vi "Ball Fight.vi"() -> ()   [LabVIEW 2014]
panel:
  in  "?":bool
  in  "Computer?":bool=TRUE
  out "BOT":u8(slide)
  out "Player":u8(slide) scale=0.0..5.0
  out "力道":dbl(slide)
  in  "pok2":bool
  out "角度":dbl(knob)
  in  "aok2":bool
  out "cannonball 2":bool
  out "角度":dbl(knob) scale=0.0..1.5
  in  "aok1":bool
  out "Wind":dbl(slide) scale=-50.0..50.0
  out "力道":dbl(slide) scale=0.0..150.0
  in  "pok1":bool
  out "cannonball":bool
  # "Angle off?"
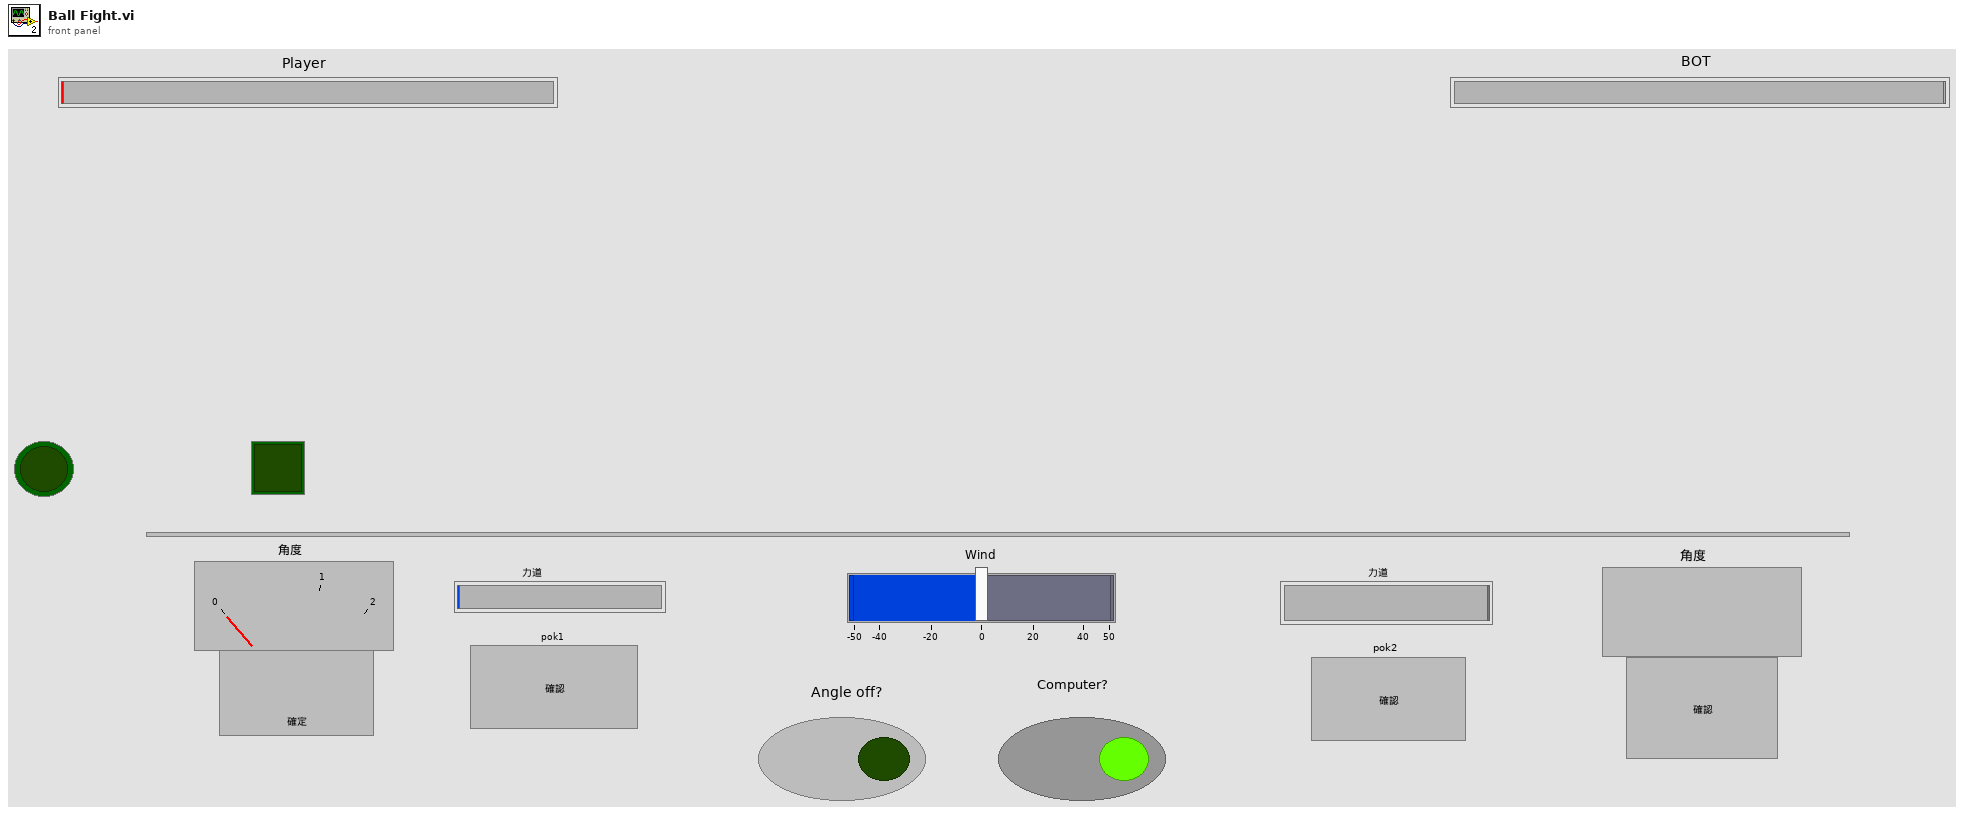
[diagram p1: front panel]
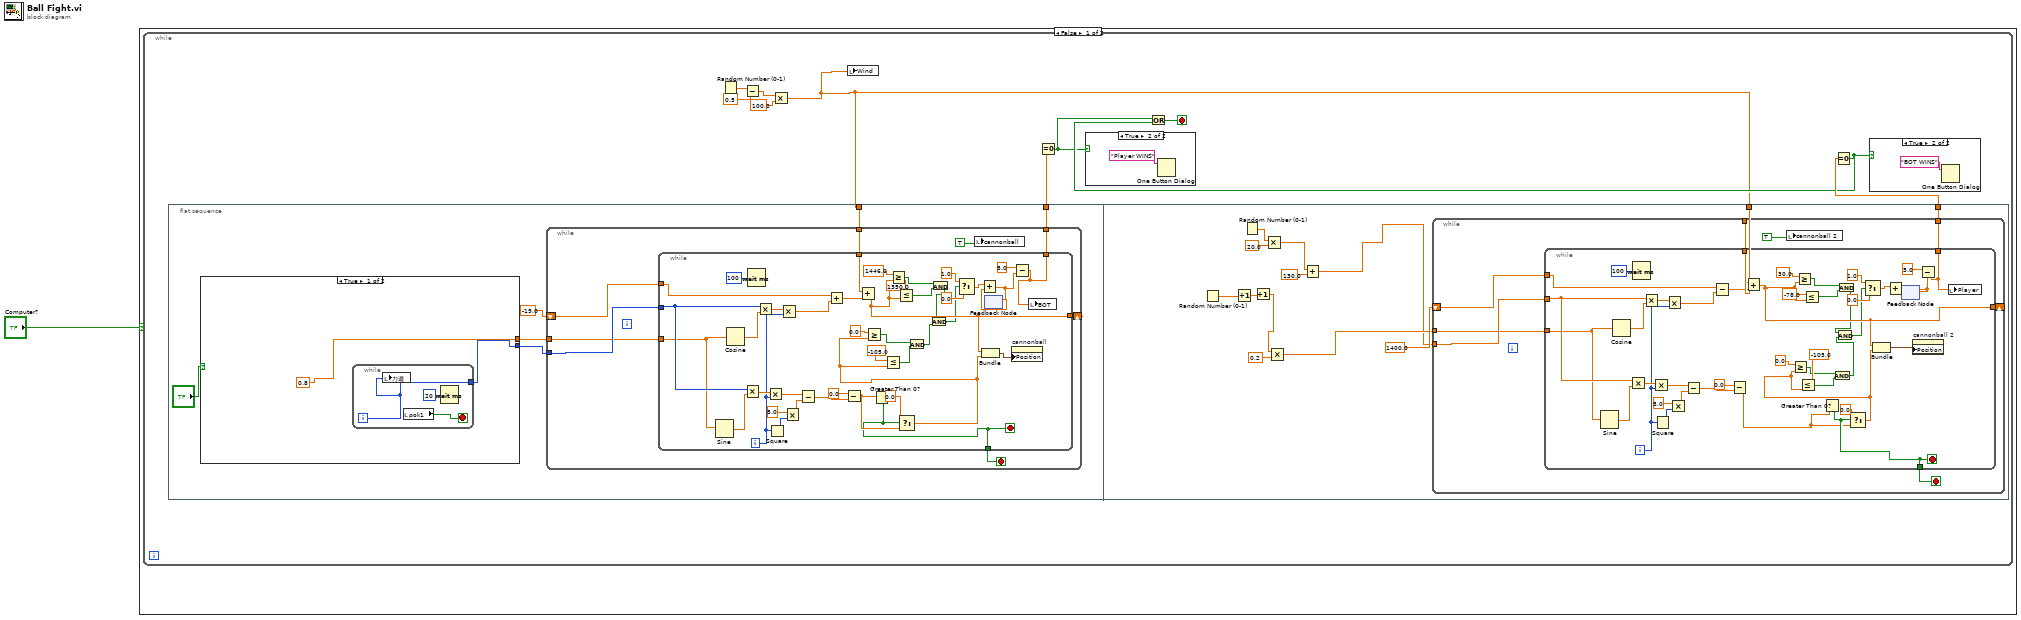
[diagram p0: block diagram]
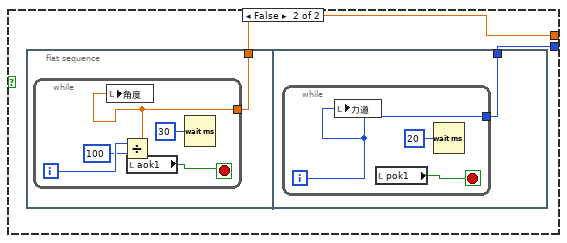
[diagram p4: hidden frame]
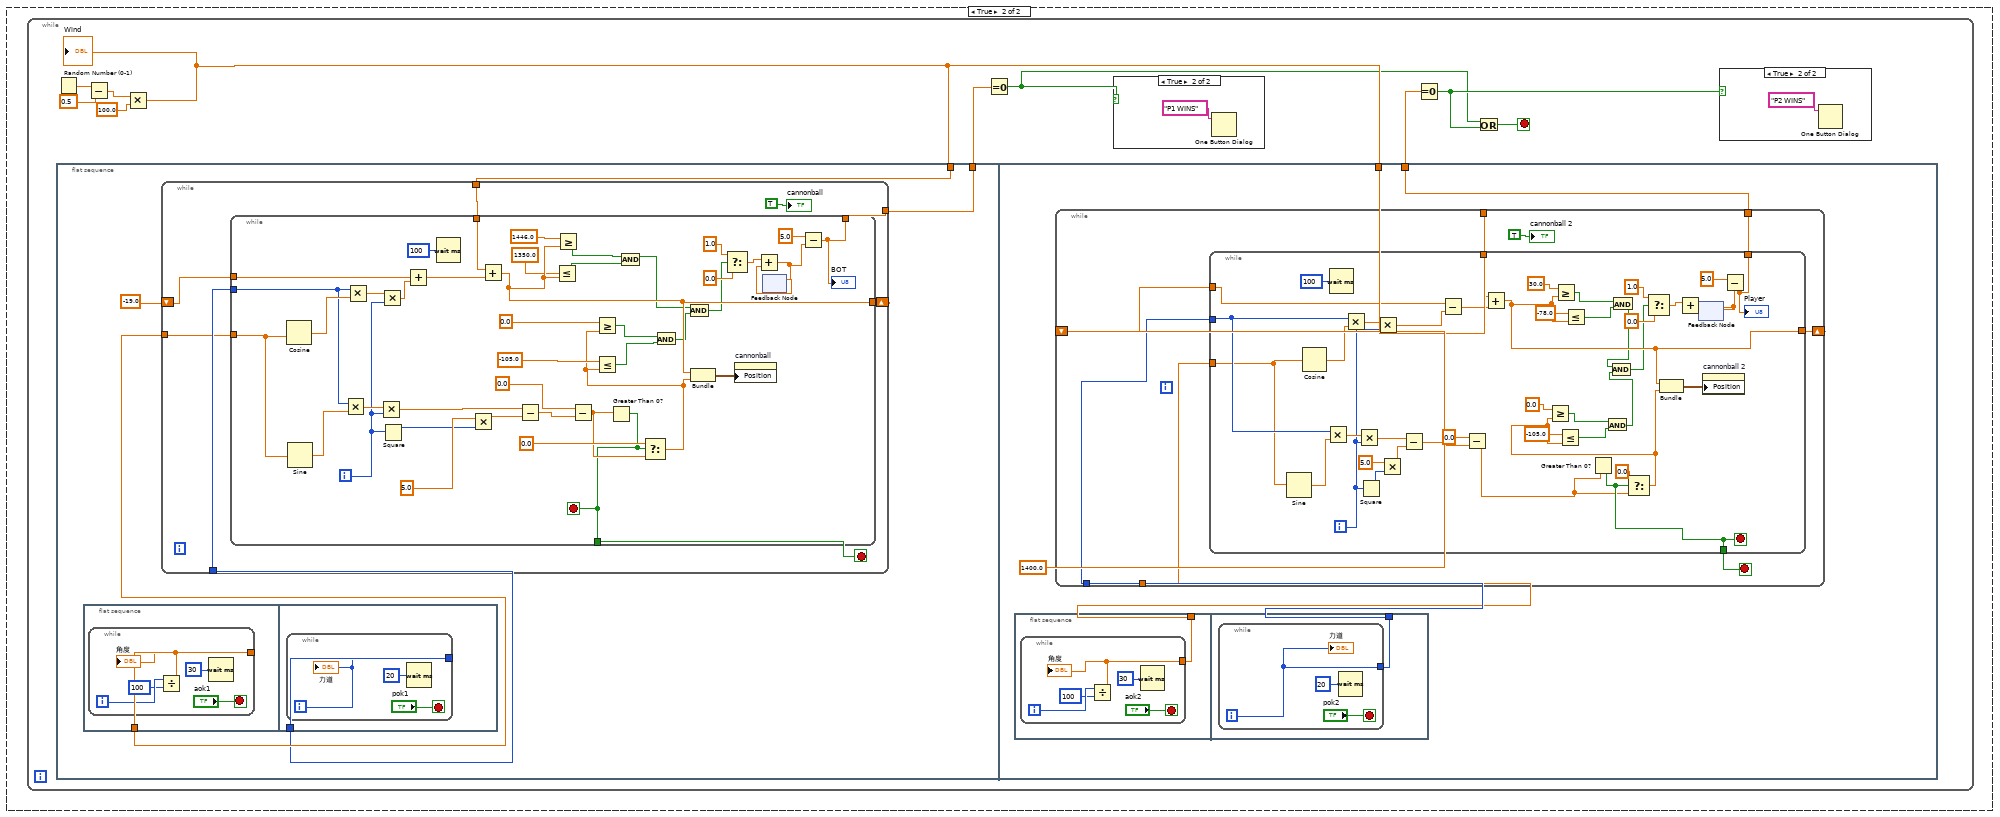
[diagram p5: hidden frame]
diagram:
  n1 = case shown="False" "Computer?" {
    frame False {
      n2 = while {
        stop <- w5 stop-if-true
        n3 = flat-sequence {
          tunnel: w2 -> [w18]
          tunnel: [w15] -> w7
          tunnel: w2 -> [w98]
          tunnel: [w97] -> w6
          frame #0 {
            n4 = case shown="True" "?" {
              tunnel: [0.8 w26] -> w17
              tunnel: [w21 w25] -> w16
              frame True {
                n5 = while {
                  tunnel: [w23] -> w21
                  i -> [w23]
                  stop <- w22 stop-if-true
                  n6 = local write "力道"(w23) -> ()
                  n7 = local read "pok1"() -> (w22:bool)
                  n8 = Wait (ms)(milliseconds to wait=u32 20) -> ()  [unwired: 1 out]
                }
              }
              frame False {
                n9 = flat-sequence {
                  tunnel: [w27] -> w26
                  tunnel: [w33] -> w25
                  frame #0 {
                    n10 = while {
                      tunnel: [w29] -> w27
                      i -> [w31]
                      stop <- w28 stop-if-true
                      n11 = Divide(x=w31, y=100) -> (x/y=w29:dbl)
                      n12 = local write "角度"(w29) -> ()
                      n13 = local read "aok1"() -> (w28:bool)
                      n14 = Wait (ms)(milliseconds to wait=u32 30) -> ()  [unwired: 1 out]
                    }
                  }
                  frame #1 {
                    n15 = while {
                      tunnel: [w35] -> w33
                      i -> [w35]
                      stop <- w34 stop-if-true
                      n16 = local write "力道"(w35) -> ()
                      n17 = local read "pok1"() -> (w34:bool)
                      n18 = Wait (ms)(milliseconds to wait=u32 20) -> ()  [unwired: 1 out]
                    }
                  }
                }
              }
            }
            n19 = while {
              shift-right: [w44] -> _
              shift-left: -19.0 -> [w43]
              tunnel: w16 -> [w42]
              tunnel: w18 -> [w40]
              tunnel: w17 -> [w39]
              tunnel: [w38] -> w15
              stop <- w41 stop-if-true
              n20 = while {
                tunnel: w42 -> [w72]
                tunnel: [w64] -> w44
                tunnel: w43 -> [w70]
                tunnel: [w69] -> w41
                tunnel: w40 -> [w67]
                tunnel: w39 -> [w66]
                tunnel: [w51] -> w38
                i -> [w79]
                stop <- w69 stop-if-true
                n21 = Sine(x=w66) -> (sin(x)=w83:dbl)
                n22 = Cosine(x=w66) -> (cos(x)=w86:dbl)
                n23 = Multiply(x=w72, y=w83) -> (x*y=w84:dbl)
                n24 = Wait (ms)(milliseconds to wait=u32 100) -> ()  [unwired: 1 out]
                n25 = Multiply(x=w72, y=w86) -> (x*y=w85:dbl)
                n26 = Multiply(x=w84, y=w79) -> (x*y=w82:dbl)
                n27 = Square(x=w79) -> (x^2=w80:i32)
                n28 = Multiply(x=w85, y=w79) -> (x*y=w71:dbl)
                n29 = Multiply(x=5.0, y=w80) -> (x*y=w78:dbl)
                n30 = Subtract(x=w82, y=w78) -> (x-y=w76:dbl)
                n31 = Add(x=w70, y=w71) -> (x+y=w68:dbl)
                n32 = Subtract(x=0.0, y=w76) -> (x-y=w73:dbl)
                n33 = Add(x=w67, y=w68) -> (x+y=w64:dbl)
                n34 = Greater Than 0?(x=w73) -> (x > 0?=w69:bool)
                n35 = Greater Or Equal?(x=1446.0, y=w64) -> (x >= y?=w62:bool)
                n36 = Less Or Equal?(x=1350.0, y=w64) -> (x <= y?=w61:bool)
                n37 = Select(t=0.0, s=w69, f=w73) -> (s? t:f=w45:dbl)
                n38 = Greater Or Equal?(x=0.0, y=w45) -> (x >= y?=w48:bool)
                n39 = Less Or Equal?(x=-105.0, y=w45) -> (x <= y?=w47:bool)
                n40 = And(x=w48, y=w47) -> (x .and. y?=w46:bool)
                n41 = And(x=w62, y=w61) -> (x .and. y?=w54:bool)
                n42 = And(x=w54, y=w46) -> (x .and. y?=w53:bool)
                n43 = Select(t=1.0, s=w53, f=0.0) -> (s? t:f=w58:dbl)
                n44 = Bundle(w64, "t"=w45) -> (w52:cluster{dbl, "t":dbl})  [unwired: 1 in]
                n45 = feedback #1() -> (w57:dbl)  [unwired: 1 in]
                n46 = Add(x=w58, y=w57) -> (x+y=w55:dbl)
                n47 = feedback-in #1(w55) -> ()
                n48 = property on="cannonball" class="Bool (strict)"("Position"=w52) -> ()  [unwired: 2 in, 2 out]
                n49 = Subtract(x=5.0, y=w55) -> (x-y=w51:dbl)
                n50 = local write "BOT"(w51) -> ()
              }
              n51 = local write "cannonball"(TRUE) -> ()
            }
          }
          frame #1 {
            n52 = Random Number (0-1)() -> (number: 0 to 1=w94:dbl)
            n53 = Increment(x=w94) -> (x+1=w93:dbl)
            n54 = Random Number (0-1)() -> (number: 0 to 1=w95:dbl)
            n55 = Increment(x=w93) -> (x+1=w91:dbl)
            n56 = Multiply(x=w95, y=20.0) -> (x*y=w87:dbl)
            n57 = Multiply(x=w91, y=0.2) -> (x*y=w90:dbl)
            n58 = Add(x=w87, y=130.0) -> (x+y=w88:dbl)
            n59 = while {
              shift-right: [w107] -> _
              shift-left: 1400.0 -> [w106]
              tunnel: w88 -> [w105]
              tunnel: w98 -> [w103]
              tunnel: w90 -> [w102]
              tunnel: [w101] -> w97
              stop <- w104 stop-if-true
              n60 = while {
                tunnel: w105 -> [w136]
                tunnel: [w121] -> w107
                tunnel: w106 -> [w134]
                tunnel: [w133] -> w104
                tunnel: w103 -> [w131]
                tunnel: w102 -> [w130]
                tunnel: [w108] -> w101
                i -> [w142]
                stop <- w133 stop-if-true
                n61 = Sine(x=w130) -> (sin(x)=w146:dbl)
                n62 = Cosine(x=w130) -> (cos(x)=w149:dbl)
                n63 = Multiply(x=w136, y=w146) -> (x*y=w147:dbl)
                n64 = Wait (ms)(milliseconds to wait=u32 100) -> ()  [unwired: 1 out]
                n65 = Multiply(x=w136, y=w149) -> (x*y=w148:dbl)
                n66 = Multiply(x=w147, y=w142) -> (x*y=w145:dbl)
                n67 = Square(x=w142) -> (x^2=w143:i32)
                n68 = Multiply(x=w148, y=w142) -> (x*y=w135:dbl)
                n69 = Multiply(x=5.0, y=w143) -> (x*y=w141:dbl)
                n70 = Subtract(x=w145, y=w141) -> (x-y=w139:dbl)
                n71 = Subtract(x=w134, y=w135) -> (x-y=w132:dbl)
                n72 = Subtract(x=0.0, y=w139) -> (x-y=w114:dbl)
                n73 = Add(x=w131, y=w132) -> (x+y=w121:dbl)
                n74 = Greater Or Equal?(x=30.0, y=w121) -> (x >= y?=w127:bool)
                n75 = Less Or Equal?(x=-78.0, y=w121) -> (x <= y?=w126:bool)
                n76 = Greater Than 0?(x=w114) -> (x > 0?=w133:bool)
                n77 = And(x=w127, y=w126) -> (x .and. y?=w112:bool)
                n78 = Select(t=0.0, s=w133, f=w114) -> (s? t:f=w110:dbl)
                n79 = Greater Or Equal?(x=0.0, y=w110) -> (x >= y?=w116:bool)
                n80 = Less Or Equal?(x=-105.0, y=w110) -> (x <= y?=w115:bool)
                n81 = And(x=w116, y=w115) -> (x .and. y?=w111:bool)
                n82 = And(x=w112, y=w111) -> (x .and. y?=w113:bool)
                n83 = Select(t=1.0, s=w113, f=0.0) -> (s? t:f=w123:dbl)
                n84 = Bundle(w121, "t"=w110) -> (w109:cluster{dbl, "t":dbl})  [unwired: 1 in]
                n85 = feedback #2() -> (w119:dbl)  [unwired: 1 in]
                n86 = Add(x=w123, y=w119) -> (x+y=w120:dbl)
                n87 = feedback-in #2(w120) -> ()
                n88 = property on="cannonball 2" class="Bool (strict)"("Position"=w109) -> ()  [unwired: 2 in, 2 out]
                n89 = Subtract(x=5.0, y=w119) -> (x-y=w108:dbl)
                n90 = local write "Player"(w108) -> ()
              }
              n91 = local write "cannonball 2"(TRUE) -> ()
            }
          }
        }
        n92 = Random Number (0-1)() -> (number: 0 to 1=w11:dbl)
        n93 = Subtract(x=w11, y=0.5) -> (x-y=w10:dbl)
        n94 = Multiply(x=w10, y=100.0) -> (x*y=w2:dbl)
        n95 = local write "Wind"(w2) -> ()
        n96 = Equal To 0?(x=w7) -> (x = 0?=w3:bool)
        n97 = case shown="True" w3 {
          frame False {
          }
          frame True {
            n98 = One Button Dialog(message="Player WINS" ("String")) -> ()  [unwired: 1 in, 1 out]
          }
        }
        n99 = Equal To 0?(x=w6) -> (x = 0?=w4:bool)
        n100 = Or(x=w3, y=w4) -> (x .or. y?=w5:bool)
        n101 = case shown="True" w4 {
          frame False {
          }
          frame True {
            n102 = One Button Dialog(message="BOT WINS" ("String")) -> ()  [unwired: 1 in, 1 out]
          }
        }
      }
    }
    frame True {
      n103 = while {
        stop <- w152 stop-if-true
        n104 = Random Number (0-1)() -> (number: 0 to 1=w159:dbl)
        n105 = flat-sequence {
          tunnel: w155 -> [w165]
          tunnel: [w162] -> w154
          tunnel: w155 -> [w229]
          tunnel: [w227] -> w153
          frame #0 {
            n106 = flat-sequence {
              tunnel: [w167] -> w164
              tunnel: [w173] -> w163
              frame #0 {
                n107 = while {
                  tunnel: [w169] -> w167
                  i -> [w170]
                  stop <- "aok1" stop-if-true
                  n108 = Divide(x=w170, y=100) -> (x/y=w169:dbl)
                  "角度" <- w169
                  n109 = Wait (ms)(milliseconds to wait=u32 30) -> ()  [unwired: 1 out]
                }
              }
              frame #1 {
                n110 = while {
                  tunnel: [w175] -> w173
                  i -> [w175]
                  stop <- "pok1" stop-if-true
                  n111 = Wait (ms)(milliseconds to wait=u32 20) -> ()  [unwired: 1 out]
                  "力道" <- w175
                }
              }
            }
            n112 = while {
              shift-right: [w184] -> _
              shift-left: -19.0 -> [w177]
              tunnel: w163 -> [w182]
              tunnel: w165 -> [w180]
              tunnel: w164 -> [w179]
              tunnel: [w178] -> w162
              stop <- w181 stop-if-true
              n113 = while {
                tunnel: w182 -> [w212]
                tunnel: [w203] -> w184
                tunnel: w177 -> [w210]
                tunnel: [w208] -> w181
                tunnel: w180 -> [w206]
                tunnel: w179 -> [w205]
                tunnel: [w193] -> w178
                i -> [w219]
                stop <- w208 stop-if-true
                n114 = Cosine(x=w205) -> (cos(x)=w226:dbl)
                n115 = Sine(x=w205) -> (sin(x)=w223:dbl)
                n116 = Multiply(x=w212, y=w223) -> (x*y=w224:dbl)
                n117 = Multiply(x=w212, y=w226) -> (x*y=w225:dbl)
                n118 = Multiply(x=w224, y=w219) -> (x*y=w222:dbl)
                n119 = Multiply(x=w225, y=w219) -> (x*y=w211:dbl)
                n120 = Square(x=w219) -> (x^2=w220:i32)
                n121 = Add(x=w210, y=w211) -> (x+y=w207:dbl)
                n122 = Wait (ms)(milliseconds to wait=u32 100) -> ()  [unwired: 1 out]
                n123 = Multiply(x=5.0, y=w220) -> (x*y=w218:dbl)
                n124 = Add(x=w206, y=w207) -> (x+y=w203:dbl)
                n125 = Subtract(x=w222, y=w218) -> (x-y=w216:dbl)
                n126 = Less Or Equal?(x=1350.0, y=w203) -> (x <= y?=w200:bool)
                n127 = Greater Or Equal?(x=1446.0, y=w203) -> (x >= y?=w201:bool)
                n128 = Subtract(x=0.0, y=w216) -> (x-y=w213:dbl)
                n129 = Greater Than 0?(x=w213) -> (x > 0?=w208:bool)
                n130 = And(x=w201, y=w200) -> (x .and. y?=w192:bool)
                n131 = Select(t=0.0, s=w208, f=w213) -> (s? t:f=w185:dbl)
                n132 = Greater Or Equal?(x=0.0, y=w185) -> (x >= y?=w188:bool)
                n133 = Less Or Equal?(x=-105.0, y=w185) -> (x <= y?=w187:bool)
                n134 = And(x=w188, y=w187) -> (x .and. y?=w186:bool)
                n135 = And(x=w192, y=w186) -> (x .and. y?=w191:bool)
                n136 = Bundle(w203, "t"=w185) -> (w209:cluster{dbl, "t":dbl})  [unwired: 1 in]
                n137 = Select(t=1.0, s=w191, f=0.0) -> (s? t:f=w197:dbl)
                n138 = property on="cannonball" class="Bool (strict)"("Position"=w209) -> ()  [unwired: 2 in, 2 out]
                n139 = feedback #3() -> (w196:dbl)  [unwired: 1 in]
                n140 = Add(x=w197, y=w196) -> (x+y=w194:dbl)
                n141 = feedback-in #3(w194) -> ()
                n142 = Subtract(x=5.0, y=w194) -> (x-y=w193:dbl)
                "BOT" <- w193
              }
              "cannonball" <- TRUE
            }
          }
          frame #1 {
            n143 = flat-sequence {
              tunnel: [w232] -> w228
              tunnel: [w238] -> w230
              frame #0 {
                n144 = while {
                  tunnel: [w234] -> w232
                  i -> [w235]
                  stop <- "aok2" stop-if-true
                  n145 = Divide(x=w235, y=100) -> (x/y=w234:dbl)
                  "角度" <- w234
                  n146 = Wait (ms)(milliseconds to wait=u32 30) -> ()  [unwired: 1 out]
                }
              }
              frame #1 {
                n147 = while {
                  tunnel: [w240] -> w238
                  i -> [w240]
                  stop <- "pok2" stop-if-true
                  n148 = Wait (ms)(milliseconds to wait=u32 20) -> ()  [unwired: 1 out]
                  "力道" <- w240
                }
              }
            }
            n149 = while {
              shift-right: [w249] -> _
              shift-left: 1400.0 -> [w248]
              tunnel: w230 -> [w246]
              tunnel: w229 -> [w244]
              tunnel: w228 -> [w243]
              tunnel: [w242] -> w227
              stop <- w245 stop-if-true
              n150 = while {
                tunnel: w246 -> [w278]
                tunnel: [w262] -> w249
                tunnel: w248 -> [w276]
                tunnel: [w274] -> w245
                tunnel: w244 -> [w272]
                tunnel: w243 -> [w271]
                tunnel: [w259] -> w242
                i -> [w284]
                stop <- w274 stop-if-true
                n151 = Sine(x=w271) -> (sin(x)=w288:dbl)
                n152 = Cosine(x=w271) -> (cos(x)=w291:dbl)
                n153 = Multiply(x=w278, y=w288) -> (x*y=w289:dbl)
                n154 = Wait (ms)(milliseconds to wait=u32 100) -> ()  [unwired: 1 out]
                n155 = Multiply(x=w278, y=w291) -> (x*y=w290:dbl)
                n156 = Multiply(x=w289, y=w284) -> (x*y=w287:dbl)
                n157 = Square(x=w284) -> (x^2=w285:i32)
                n158 = Multiply(x=w290, y=w284) -> (x*y=w277:dbl)
                n159 = Multiply(x=5.0, y=w285) -> (x*y=w283:dbl)
                n160 = Subtract(x=w287, y=w283) -> (x-y=w281:dbl)
                n161 = Subtract(x=w276, y=w277) -> (x-y=w273:dbl)
                n162 = Subtract(x=0.0, y=w281) -> (x-y=w254:dbl)
                n163 = Add(x=w272, y=w273) -> (x+y=w262:dbl)
                n164 = Greater Or Equal?(x=30.0, y=w262) -> (x >= y?=w268:bool)
                n165 = Less Or Equal?(x=-78.0, y=w262) -> (x <= y?=w267:bool)
                n166 = Greater Than 0?(x=w254) -> (x > 0?=w274:bool)
                n167 = And(x=w268, y=w267) -> (x .and. y?=w252:bool)
                n168 = Select(t=0.0, s=w274, f=w254) -> (s? t:f=w250:dbl)
                n169 = Greater Or Equal?(x=0.0, y=w250) -> (x >= y?=w256:bool)
                n170 = Less Or Equal?(x=-105.0, y=w250) -> (x <= y?=w255:bool)
                n171 = And(x=w256, y=w255) -> (x .and. y?=w251:bool)
                n172 = And(x=w252, y=w251) -> (x .and. y?=w253:bool)
                n173 = Select(t=1.0, s=w253, f=0.0) -> (s? t:f=w264:dbl)
                n174 = Bundle(w262, "t"=w250) -> (w275:cluster{dbl, "t":dbl})  [unwired: 1 in]
                n175 = feedback #4() -> (w260:dbl)  [unwired: 1 in]
                n176 = Add(x=w264, y=w260) -> (x+y=w261:dbl)
                n177 = feedback-in #4(w261) -> ()
                n178 = property on="cannonball 2" class="Bool (strict)"("Position"=w275) -> ()  [unwired: 2 in, 2 out]
                n179 = Subtract(x=5.0, y=w260) -> (x-y=w259:dbl)
                "Player" <- w259
              }
              "cannonball 2" <- TRUE
            }
          }
        }
        n180 = Subtract(x=w159, y=0.5) -> (x-y=w158:dbl)
        n181 = Multiply(x=w158, y=100.0) -> (x*y=w155:dbl)
        "Wind" <- w155
        n182 = Equal To 0?(x=w154) -> (x = 0?=w150:bool)
        n183 = case shown="True" w150 {
          frame False {
          }
          frame True {
            n184 = One Button Dialog(message="P1 WINS" ("String")) -> ()  [unwired: 1 in, 1 out]
          }
        }
        n185 = Equal To 0?(x=w153) -> (x = 0?=w151:bool)
        n186 = Or(x=w150, y=w151) -> (x .or. y?=w152:bool)
        n187 = case shown="True" w151 {
          frame False {
          }
          frame True {
            n188 = One Button Dialog(message="P2 WINS" ("String")) -> ()  [unwired: 1 in, 1 out]
          }
        }
      }
    }
  }
